vi "parce_string_to_elements_recursively.vi"(8 "error in (no error)":errorcluster, 11 "BSONdoc":u8[](array[numeric])) -> (0 "error out":errorcluster, 3 "arrayOfElements":T1[](array[typedef]))   [LabVIEW 2015, in "BSON_convertors_Library.lvlib"]
uses:
  BSON_convertors_Library.lvlib
  typedefs/BSONelement.ctl
  typedefs/dataType.ctl
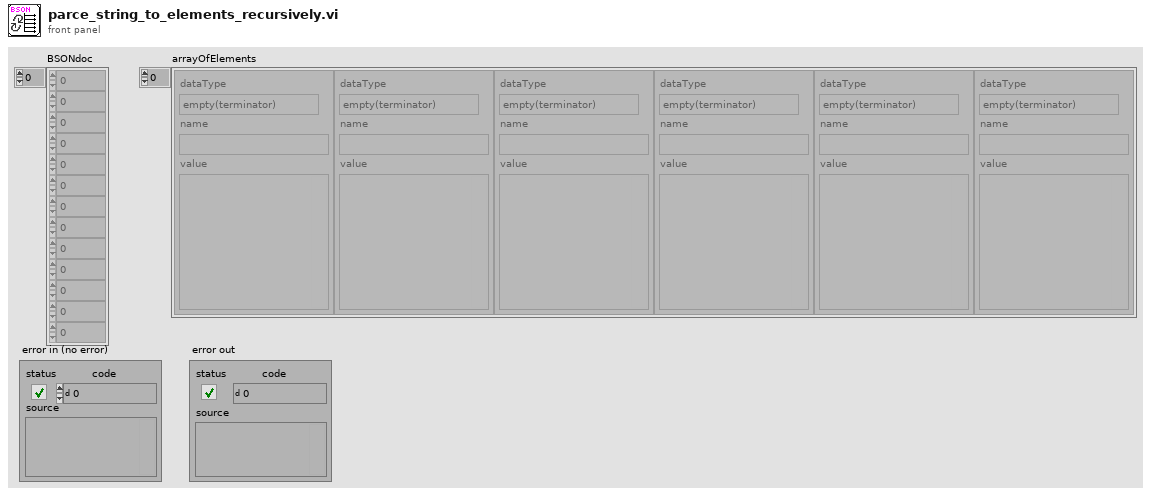
[diagram p1: front panel]
types:
  T1 = typedef "BSON_convertors_Library.lvlib/BSONelement.ctl" = cluster{"dataType":T2, "name":string, "value":variant}
  T2 = typedef "BSON_convertors_Library.lvlib/dataType.ctl" = enum8{"empty(terminator)", "double", "string", "document", "array", "binary", "Deprecated(Undefined)", "ObjectId", "boolean", "UTC datetime", "Null value", "cstring", "Deprecated(DBPointer)", "JavaScript", "Deprecated(Symbol)", "code_w_s", "int32", "uint64", "int64", "ext (decimal128)", "Min key", "Max key"}
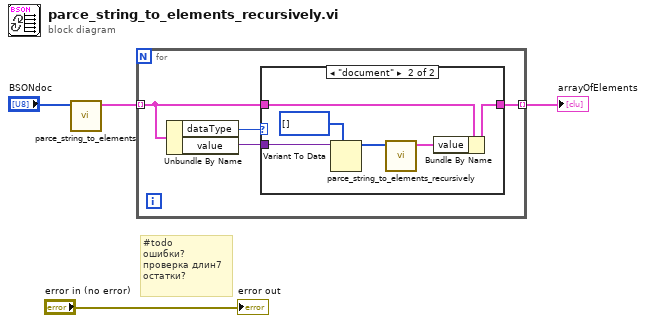
[diagram p0: block diagram]
diagram:
  # "#todo \nошибки?\nпроверка длин7\nостатки?"
  n1 = call "parce_string_to_elements.vi"("BSONbytes"="BSONdoc") -> ("arrayOfElements"=w3:T1[])  [unwired: 8 in, 2 out]
  n2 = for {
    tunnel: w3 -> [w6] mode=indexing
    tunnel: [w5] -> w4 mode=indexing
    n3 = Unbundle By Name(w6) -> ("dataType"=w8:T2, "value"=w7:variant)
    n4 = case shown="\"document\"" w8 {
      tunnel: w7 -> [_ w15]
      tunnel: w6 -> [w9 w12]
      tunnel: [w9 w10] -> w5
      frame Default {
      }
      frame "document" {
        n5 = Variant To Data(type=u8[] [], Variant=w15) -> (data=w13:u8[])  [unwired: 1 in, 1 out]
        n6 = call "parce_string_to_elements_recursively.vi"("BSONdoc"=w13) -> ("arrayOfElements"=w11:T1[])  [unwired: 9 in, 1 out]
        n7 = Bundle By Name(cluster=w12, "value"=w11) -> (w10:T1)
      }
    }
  }
  "arrayOfElements" <- w4
  "error out" <- "error in (no error)"
